vi "Get Components.vi"(8 "error in":errorcluster, 11 "DAQ Board in":refnum<class "DAQ Board Design.lvclass">) -> (0 "error out":errorcluster, 2 "components":refnum<class "Component.lvclass">[](array[class]), 3 "DAQ Board out":refnum<class "DAQ Board Design.lvclass">)   [LabVIEW 2023, in "DAQ Board Design.lvclass"]
doc: "Get an array of components for the board."
uses:
  DAQ Board Design.lvclass
  Component/Component.lvclass
  ADConverter/AD Converter.lvclass
  c:/dev/_r/4/eng/lv-core/lvpostprocessingd/lv_mc_x86_64/dist_i386/examples/Object-Oriented Programming/Board Testing/Object Design/Component/Component.lvclass
  DAConverter/DA Converter.lvclass
  FPGAChip/FPGA Chip.lvclass
  Board/Component Orientation and Position.ctl
  Resistor/Resistor.lvclass
  Board/Board Design.lvclass
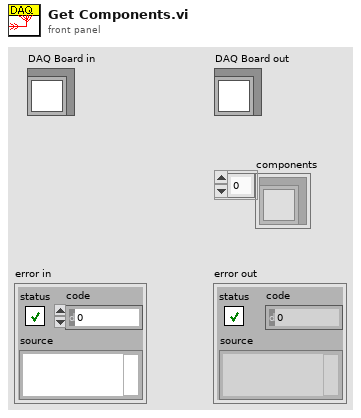
[diagram p1: front panel]
types:
  T1 = typedef "Board Design.lvclass/Component Orientation and Position.ctl" = cluster{"row":i16, "column":i16, "landscape?":bool}
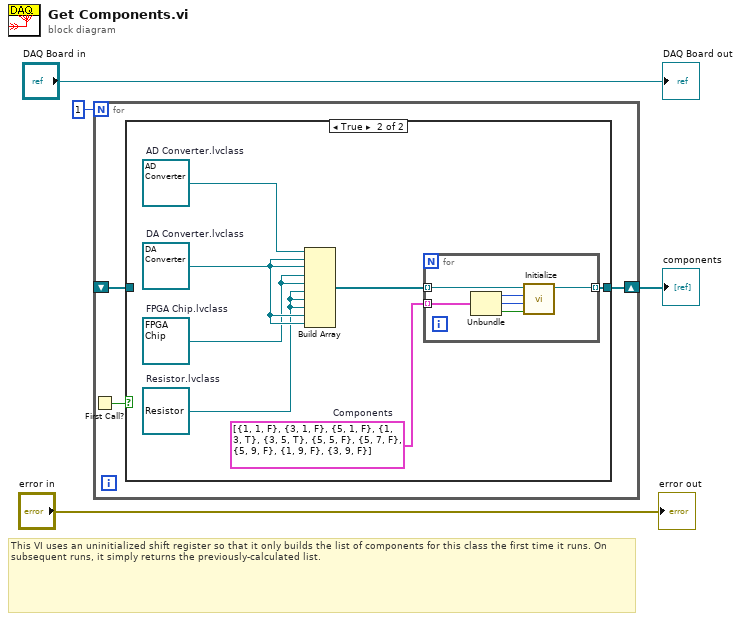
[diagram p0: block diagram]
diagram:
  # "This VI uses an uninitialized shift register so that it only builds the list of components for this class the first time it runs. On subsequent runs, it simply returns the previously-calculated list."
  n1 = for {
    N: 1 -> [_]
    shift-right: [w7] -> w2
    shift-left: _ -> [w5]
    n2 = First Call?() -> (First Call?: T/F=w6:bool)
    n3 = case shown="True" w6 {
      tunnel: [w8 w14] -> w7
      tunnel: w5 -> [w8 _]
      frame False {
      }
      frame True {
        w10 = refnum<class "Resistor.lvclass"> refnum  # Resistor.lvclass
        w13 = T1[] [{"row"=1, "column"=1, "landscape?"=FALSE}, {"row"=3, "column"=1, "landscape?"=FALSE}, {"row"=5, "column"=1, "landscape?"=FALSE}, {"row"=1, "column"=3, "landscape?"=TRUE}, {"row"=3, "column"=5, "landscape?"=TRUE}, {"row"=5, "column"=5, "landscape?"=FALSE}, {"row"=5, "column"=7, "landscape?"=FALSE}, {"row"=5, "column"=9, "landscape?"=FALSE}, {"row"=1, "column"=9, "landscape?"=FALSE}, {"row"=3, "column"=9, "landscape?"=FALSE}]  # Components
        w9 = refnum<class "FPGA Chip.lvclass"> refnum  # FPGA Chip.lvclass
        w11 = refnum<class "DA Converter.lvclass"> refnum  # DA Converter.lvclass
        w12 = refnum<class "AD Converter.lvclass"> refnum  # AD Converter.lvclass
        n4 = Build Array(w12, w11, w11, w9, w9, w10, w10, w10, w11, w11) -> (w15:refnum<class "Component.lvclass">[])
        n5 = for {
          tunnel: w15 -> [w21] mode=indexing
          tunnel: [w20] -> w14 mode=indexing
          tunnel: w13 -> [w19] mode=indexing
          n6 = Unbundle(w19) -> ("row"=w18:i16, "column"=w17:i16, "landscape?"=w16:bool)
          n7 = call "Initialize.vi"("landscape?"=w16, "column"=w17, "row"=w18, "Component.lvclass in"=w21) -> ("Component.lvclass out"=w20:refnum<class "Component.lvclass">)  [unwired: 7 in]
        }
      }
    }
  }
  "components" <- w2
  "error out" <- "error in"
  "DAQ Board out" <- "DAQ Board in"
